vi "onStart.vi"(8 "error in (no error)":errorcluster, 11 "MAUI":refnum<class "MAUI.lvclass">) -> (0 "error out":errorcluster, 3 "MAUI out":refnum<class "MAUI.lvclass">)   [LabVIEW 2019, in "MAUI.lvclass"]
doc: "JKI State Machine Objects (SMO) 1.3.0.56\nJKI - JKI\nCopyright (c) 2017, JKI"
uses:
  MAUI.lvclass
  <userlib>/LevyLab/Embedded UI/SMO.UI.Embedded/Embedded UI.lvclass
  C:/Program Files (x86)/National Instruments/LabVIEW 2019/vi.lib/JKI/JKI SMO/SMO/SMO.lvclass
  MAUI.lvclass/MAUI.ctl
  <vilib>/JKI/JKI SMO/SMO.UI/SMO.UI.lvclass
  <vilib>/JKI/JKI SMO/SMO/SMO.lvclass
panel:
  # "For instructions on how to use the JKI State Machine Objects, examples and video tutorials, visit:\nhttp://jki.net/state-machine-objects/\n\nJKI State Machine Objects™\nhttp://jki.net/state-machine-objects/\nCopyright (C) 2005-2015, JKI <info@jki.net>\nALL RIGHTS RESERVED"
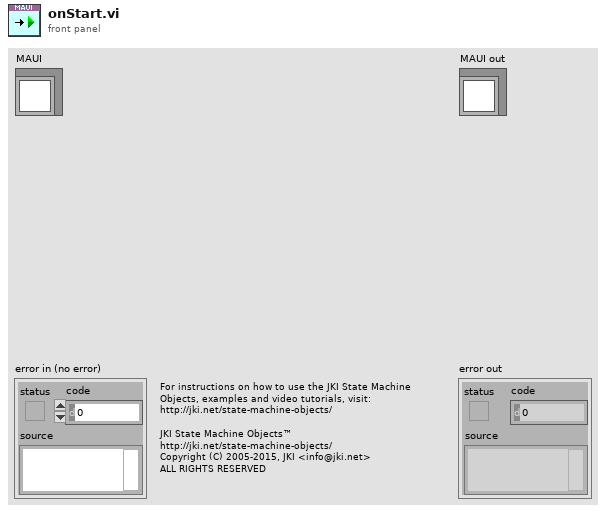
[diagram p1: front panel]
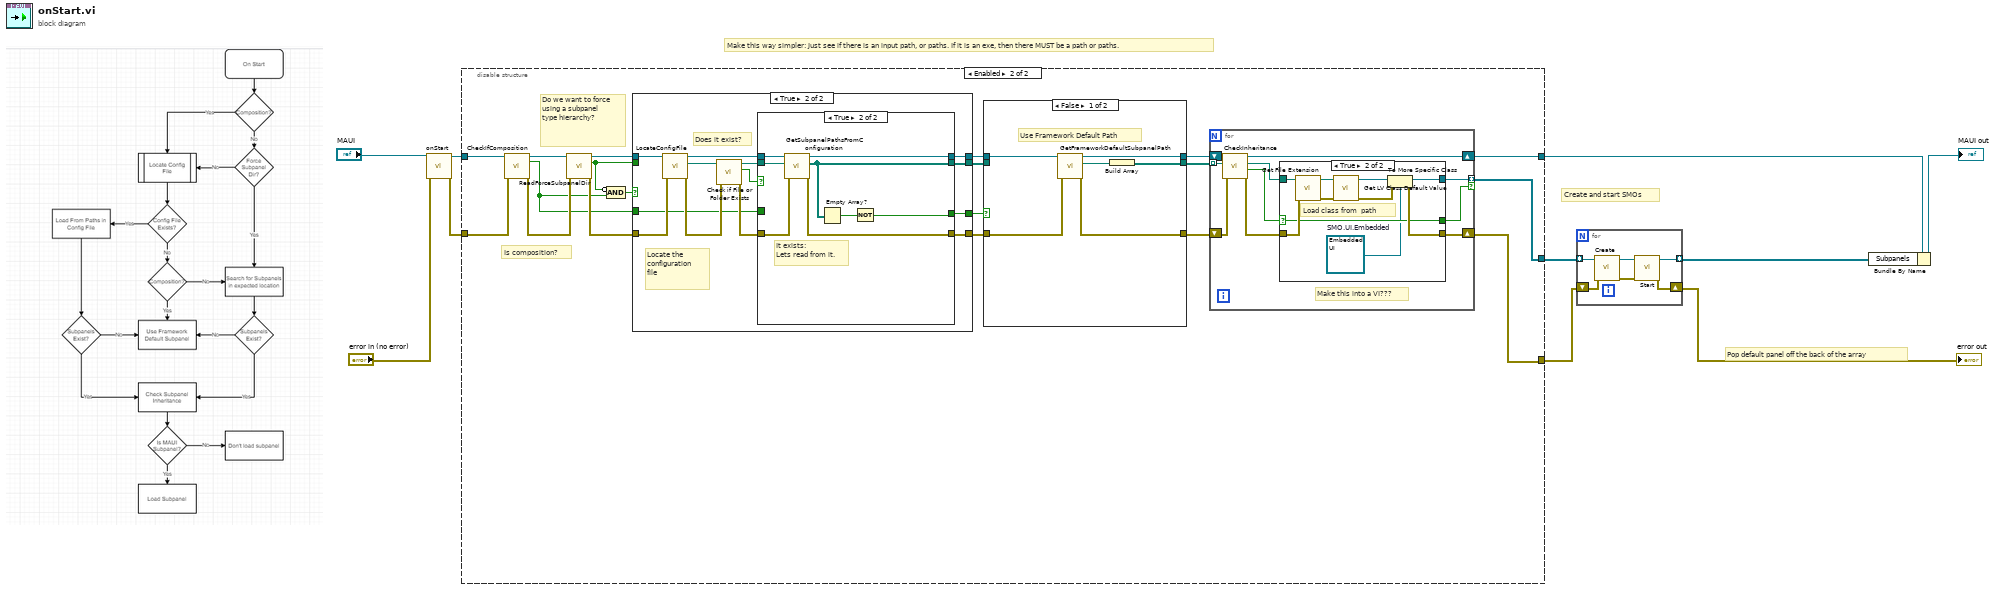
[diagram p0: block diagram]
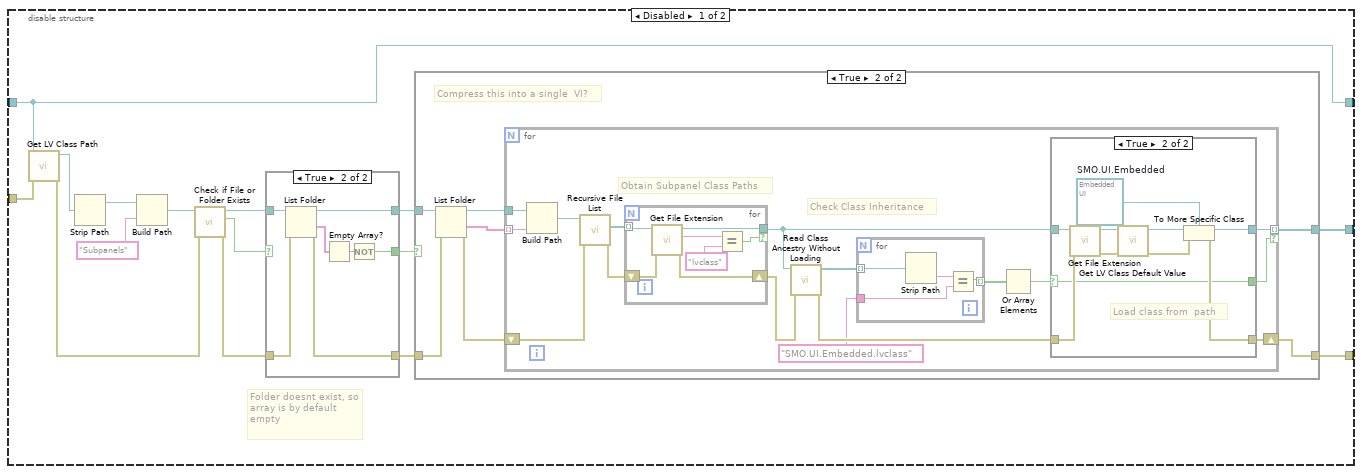
[diagram p2: hidden frame]
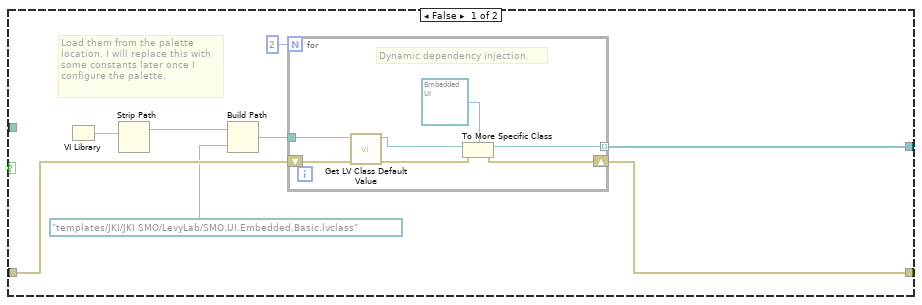
[diagram p4: hidden frame]
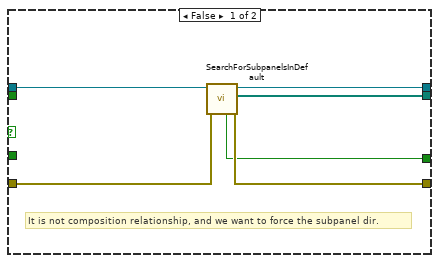
[diagram p8: hidden frame]
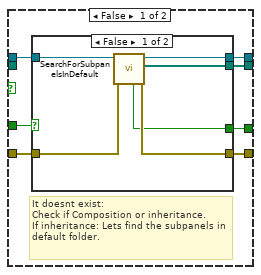
[diagram p9: hidden frame]
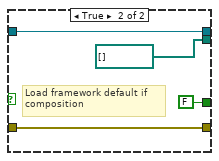
[diagram p10: hidden frame]
diagram:
  # "Make this way simpler: Just see if there is an input path, or paths. If it is an exe, then there MUST be a path or paths."
  # "Create and start SMOs"
  # "Pop default panel off the back of the array"
  n1 = call-parent "onStart.vi"("error in (no error)"="error in (no error)", "SMO"="MAUI") -> ("error out"=w10:errorcluster, "SMO out"=w3:refnum<class "MAUI.lvclass">)  [unwired: 8 in]
  n2 = disable-structure "Diagram Disable Structure" shown="Enabled" {
    disable-tunnel: w10 -> [w24 w113]
    disable-tunnel: [w16 w98] -> w6
    disable-tunnel: [w21 w100] -> w7
    disable-tunnel: w3 -> [w11 w97]
    disable-tunnel: [w11 w99] -> w2
    frame Disabled {
      # "Folder doesnt exist, so array is by default empty"
      n3 = call <vilib>:"Get LV Class Path.vi"("error in (no error)"=w24, "object"=w11) -> ("error out"=w25:errorcluster, "class path"=w20:path)  [unwired: 8 in]
      n4 = Strip Path(path=w20) -> (stripped path=w19:path)  [unwired: 1 out]
      n5 = Build Path(base path=w19, name or relative path="Subpanels") -> (appended path=w17:path)
      n6 = call <vilib>:"Check if File or Folder Exists.vi"("error in (no error)"=w25, "path"=w17) -> ("error out"=w23:errorcluster, "file or folder exists?"=w14:bool, "dup path"=w15:path)  [unwired: 7 in]
      n7 = case shown="True" w14 {
        selector: w14 -> [w27 _]
        tunnel: w15 -> [w26 w33]
        tunnel: w23 -> [w28 w35]
        tunnel: [w28 w34] -> w22
        tunnel: [w27 w31] -> w13
        tunnel: [w26 w29] -> w12
        frame False {
        }
        frame True {
          n8 = List Folder(path=w33, error in=w35) -> (path out=w29:path, folder names=w30:string[], error out=w34:errorcluster)  [unwired: 2 in, 1 out]
          n9 = Empty Array?(array=w30) -> (empty?=w32:bool)
          n10 = Not(x=w32) -> (.not. x?=w31:bool)
        }
      }
      n11 = case shown="True" w13 {
        tunnel: w12 -> [_ w54]
        tunnel: w22 -> [w42 w56]
        tunnel: [w43 w55] -> w21
        tunnel: [w36 w51] -> w16
        frame False {
          # "Load them from the palette location. I will replace this with some constants later once I configure the palette."
          n12 = VI Library() -> (path=w41:path)
          n13 = Strip Path(path=w41) -> (stripped path=w40:path)  [unwired: 1 out]
          n14 = Build Path(base path=w40, name or relative path=path "templates/JKI/JKI SMO/LevyLab/SMO.UI.Embedded.Basic.lvclass") -> (appended path=w37:path)
          n15 = for {
            N: 2 -> [_]
            tunnel: w37 -> [w47]
            shift-right: [w49] -> w43
            shift-left: w42 -> [w50]
            tunnel: [w46] -> w36 mode=indexing
            # "Dynamic dependency injection."
            n16 = call <vilib>:"Get LV Class Default Value.vi"("error in (no error)"=w50, "class path"=w47) -> ("error out"=w48:errorcluster, "object"=w44:refnum<class>)  [unwired: 8 in]
            n17 = To More Specific Class(target class=refnum<class "Embedded UI.lvclass"> refnum ("SMO.UI.Embedded"), reference=w44, error in=w48) -> (specific class reference=w46:refnum<class "Embedded UI.lvclass">, error out=w49:errorcluster)
          }
        }
        frame True {
          # "Compress this into a single  VI?"
          n18 = List Folder(path=w54, error in=w56) -> (path out=w53:path, folder names=w52:string[], error out=w57:errorcluster)  [unwired: 2 in, 1 out]
          n19 = for {
            tunnel: w53 -> [w68]
            tunnel: w52 -> [w67] mode=indexing
            tunnel: [w63] -> w51 mode=indexing if=w58
            shift-right: [w69] -> w55
            shift-left: w57 -> [w73]
            # "Check Class Inheritance"
            # "Obtain Subpanel Class Paths"
            n20 = Build Path(base path=w68, name or relative path=w67) -> (appended path=w66:path)
            n21 = call <vilib>:"Recursive File List.vi"("error in (no error)"=w73, "Folder Path"=w66) -> ("error out"=w72:errorcluster, "All Files in Dir"=w65:path[])  [unwired: 5 in, 3 out]
            n22 = for {
              tunnel: w65 -> [w92] mode=indexing
              tunnel: [w91] -> w64 if=w90
              shift-right: [w95] -> w71
              shift-left: w72 -> [w96]
              n23 = call <vilib>:"Get File Extension.vi"("error in (no error)"=w96, "file"=w92) -> ("error out"=w95:errorcluster, "lowercase file extension"=w94:string, "dup file"=w91:path)  [unwired: 5 in, 2 out]
              n24 = Equal?(x=w94, y="lvclass") -> (x = y?=w90:bool)
            }
            n25 = call <vilib>:"Read Class Ancestry Without Loading.vi"("error in (no error)"=w71, "LabVIEW Class Path"=w64) -> ("error out"=w70:errorcluster, "Class Ancestry"=w62:path[])  [unwired: 8 in]
            n26 = for {
              tunnel: w62 -> [w89] mode=indexing
              tunnel: [w87] -> w61 mode=indexing
              tunnel: "SMO.UI.Embedded.lvclass" -> [w86]
              n27 = Strip Path(path=w89) -> (name=w88:string)  [unwired: 1 out]
              n28 = Equal?(x=w88, y=w86) -> (x = y?=w87:bool)
            }
            n29 = Or Array Elements(Boolean array=w61) -> (logical OR=w59:bool)
            n30 = case shown="True" w59 {
              selector: w59 -> [w74 w77]
              tunnel: w64 -> [_ w79]
              tunnel: [_ w81] -> w63
              tunnel: w70 -> [w75 w83]
              tunnel: [w75 w84] -> w69
              tunnel: [w74 w77] -> w58
              frame False {
                # "This case gets filtered later by conditional terminals. Don't do anything here."
                # "This case gets filtered later by conditional terminals"
              }
              frame True {
                w76 = refnum<class "Embedded UI.lvclass"> refnum  # SMO.UI.Embedded
                # "Load class from  path"
                n31 = call <vilib>:"Get File Extension.vi"("error in (no error)"=w83, "file"=w79) -> ("error out"=w82:errorcluster, "dup file"=w78:path)  [unwired: 5 in, 3 out]
                n32 = call <vilib>:"Get LV Class Default Value.vi"("error in (no error)"=w82, "class path"=w78) -> ("error out"=w85:errorcluster, "object"=w80:refnum<class>)  [unwired: 8 in]
                n33 = To More Specific Class(target class=w76, reference=w80, error in=w85) -> (specific class reference=w81:refnum<class "Embedded UI.lvclass">, error out=w84:errorcluster)
              }
            }
          }
        }
      }
    }
    frame Enabled {
      # "Do we want to force using a subpanel type hierarchy?"
      # "Is composition?"
      # "Steps"
      n34 = call "CheckIfComposition.vi"("error in (no error)"=w113, "SMO.UI.MAUI in"=w97) -> ("error out"=w115:errorcluster, "Is Composition?"=w108:bool, "SMO.UI.MAUI out"=w111:refnum<class "MAUI.lvclass">)  [unwired: 7 in]
      n35 = call "ReadForceSubpanelDir.vi"("error in (no error)"=w115, "SMO.UI.MAUI in"=w111) -> ("error out"=w114:errorcluster, "ForceSubpanelDir?"=w107:bool, "SMO.UI.MAUI out"=w109:refnum<class "MAUI.lvclass">)  [unwired: 7 in]
      n36 = Compound Arithmetic op=AND(invert w107, w108) -> (w110:bool)
      n37 = case shown="True" w110 {
        tunnel: w114 -> [w151 w165]
        tunnel: [w152 w163] -> w112
        tunnel: w109 -> [w149 w161]
        tunnel: [w150 w156] -> w106
        tunnel: w108 -> [_ w155]
        tunnel: w107 -> [_ _]
        tunnel: [w148 w153] -> w104
        tunnel: [w147 w154] -> w105
        frame False {
          # "It is not composition relationship, and we want to force the subpanel dir."
          n38 = call "SearchForSubpanelsInDefault.vi"("error in (no error)"=w151, "SMO.UI.MAUI in"=w149) -> ("error out"=w152:errorcluster, "Array"=w148:path[], "SMO.UI.MAUI out"=w150:refnum<class "MAUI.lvclass">, "Subpanels Found?"=w147:bool)  [unwired: 6 in]
        }
        frame True {
          # "Does it exist?"
          # "Locate the configuration file"
          n39 = call "LocateConfigFile.vi"("error in (no error)"=w165, "SMO.UI.MAUI in"=w161) -> ("error out"=w164:errorcluster, "Config File Path"=w160:path, "SMO.UI.MAUI out"=w157:refnum<class "MAUI.lvclass">)  [unwired: 7 in]
          n40 = call <vilib>:"Check if File or Folder Exists.vi"("error in (no error)"=w164, "path"=w160) -> ("error out"=w162:errorcluster, "file or folder exists?"=w159:bool, "dup path"=w158:path)  [unwired: 7 in]
          n41 = case shown="True" w159 {
            tunnel: [w171 w190] -> w163
            tunnel: w162 -> [w172 w189]
            tunnel: w158 -> [_ w186]
            tunnel: w157 -> [w169 w187]
            tunnel: [w170 w188] -> w156
            tunnel: w155 -> [w168 _]
            tunnel: [w167 w184] -> w154
            tunnel: [w166 w183] -> w153
            frame False {
              # "It doesnt exist:\nCheck if Composition or inheritance.\nIf inheritance: Lets find the subpanels in default folder."
              n42 = case shown="False" w168 {
                tunnel: [w176 w181] -> w170
                tunnel: w169 -> [w175 w181]
                tunnel: w172 -> [w177 w182]
                tunnel: [w178 w182] -> w171
                tunnel: [w174 FALSE ("Subpanels Found?")] -> w167
                tunnel: [w173 path[] [] ("Array")] -> w166
                frame False {
                  n43 = call "SearchForSubpanelsInDefault.vi"("error in (no error)"=w177, "SMO.UI.MAUI in"=w175) -> ("error out"=w178:errorcluster, "Array"=w173:path[], "SMO.UI.MAUI out"=w176:refnum<class "MAUI.lvclass">, "Subpanels Found?"=w174:bool)  [unwired: 6 in]
                }
                frame True {
                  # "Load framework default if \ncomposition"
                }
              }
            }
            frame True {
              # "It exists:\nLets read from it."
              n44 = call "GetSubpanelPathsFromConfiguration.vi"("error in (no error)"=w189, "Path"=w186, "SMO.UI.MAUI in"=w187) -> ("error out"=w190:errorcluster, "Array"=w183:path[], "SMO.UI.MAUI out"=w188:refnum<class "MAUI.lvclass">)  [unwired: 6 in]
              n45 = Empty Array?(array=w183) -> (empty?=w185:bool)
              n46 = Not(x=w185) -> (.not. x?=w184:bool)
            }
          }
        }
      }
      n47 = case shown="False" w105 {
        tunnel: w106 -> [w142 w145]
        tunnel: [w143 w145] -> w103
        tunnel: [w139 w146] -> w101
        tunnel: w112 -> [w138 w146]
        tunnel: [w140 w144] -> w102
        tunnel: w104 -> [_ w144]
        frame False {
          # "Use Framework Default Path"
          n48 = call "GetFrameworkDefaultSubpanelPath.vi"("error in (no error)"=w138, "SMO.UI.MAUI in"=w142) -> ("error out"=w139:errorcluster, "path"=w141:path, "SMO.UI.MAUI out"=w143:refnum<class "MAUI.lvclass">)  [unwired: 7 in]
          n49 = Build Array(w141) -> (w140:path[])
        }
        frame True {
          # "Subpanels Found\nDont use framework default"
        }
      }
      n50 = for {
        tunnel: w102 -> [w124] mode=indexing
        shift-right: [w120] -> w100
        shift-left: w101 -> [w123]
        shift-right: [w122] -> w99
        shift-left: w103 -> [w125]
        tunnel: [w117] -> w98 mode=indexing if=w116
        # "Make this into a VI???"
        n51 = call "CheckInheritance.vi"("error in (no error)"=w123, "Path"=w124, "SMO.UI.MAUI in"=w125) -> ("error out"=w121:errorcluster, "IsEmbedded?"=w119:bool, "Path"=w118:path, "SMO.UI.MAUI out"=w122:refnum<class "MAUI.lvclass">)  [unwired: 5 in]
        n52 = case shown="True" w119 {
          selector: w119 -> [w126 w129]
          tunnel: w118 -> [_ w131]
          tunnel: [_ w133] -> w117
          tunnel: w121 -> [w127 w135]
          tunnel: [w127 w136] -> w120
          tunnel: [w126 w129] -> w116
          frame False {
            # "This case gets filtered later by conditional terminals. Don't do anything here."
            # "This case gets filtered later by conditional terminals"
          }
          frame True {
            w128 = refnum<class "Embedded UI.lvclass"> refnum  # SMO.UI.Embedded
            # "Load class from  path"
            n53 = call <vilib>:"Get File Extension.vi"("error in (no error)"=w135, "file"=w131) -> ("error out"=w134:errorcluster, "dup file"=w130:path)  [unwired: 5 in, 3 out]
            n54 = call <vilib>:"Get LV Class Default Value.vi"("error in (no error)"=w134, "class path"=w130) -> ("error out"=w137:errorcluster, "object"=w132:refnum<class>)  [unwired: 8 in]
            n55 = To More Specific Class(target class=w128, reference=w132, error in=w137) -> (specific class reference=w133:refnum<class "Embedded UI.lvclass">, error out=w136:errorcluster)
          }
        }
      }
    }
  }
  n56 = for {
    tunnel: w6 -> [w193] mode=indexing
    tunnel: [w192] -> w1 mode=indexing
    shift-right: [w194] -> w8
    shift-left: w7 -> [w195]
    n57 = call <vilib>:"Create.vi"("error in (no error)"=w195, "SMO"=w193) -> ("error out"=w196:errorcluster, "SMO out"=w191:refnum<class "Embedded UI.lvclass">)  [unwired: 7 in, 1 out]
    n58 = call <vilib>:"Start.vi"("error in (no error)"=w196, "SMO"=w191) -> ("error out"=w194:errorcluster, "SMO out"=w192:refnum<class "Embedded UI.lvclass">)  [unwired: 8 in]
  }
  "error out" <- w8
  n59 = Bundle By Name(cluster=w2, "Subpanels"=w1) -> (→"MAUI out":refnum<class "MAUI.lvclass">)
